vi "Destroy IntelliSenseString.vi"(0 "IntelliSense String":refnum<class "IntelliSenseStringControl.lvclass">, 11 "error in (no error)":errorcluster) -> (15 "error out":errorcluster)   [LabVIEW 2016, in "StringIntelliSense.lvlib"]
uses:
  StringIntelliSense.lvlib
  IntelliSenseStringControl.lvclass
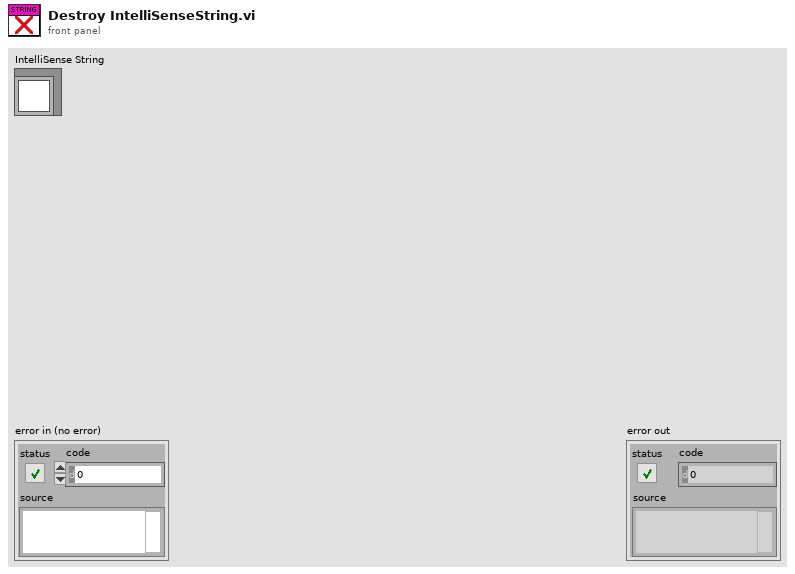
[diagram p1: front panel]
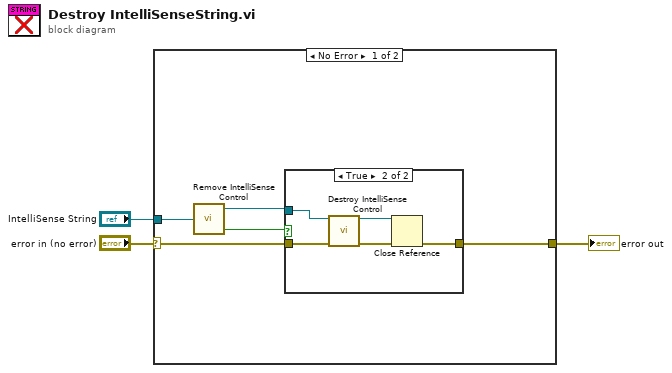
[diagram p0: block diagram]
diagram:
  n1 = case shown="No Error" "error in (no error)" {
    selector: "error in (no error)" -> [w7 w15]
    tunnel: [w8 w15] -> w2
    tunnel: "IntelliSense String" -> [w6 _]
    frame No Error {
      n2 = call "Remove IntelliSense Control.vi"("IntelliSenseStringControl"=w6) -> ("IntelliSenseStringControl"=w5:refnum<class "IntelliSenseStringControl.lvclass">, "removed?"=w4:bool)  [unwired: 1 in]
      n3 = case shown="True" w4 {
        tunnel: [w9 w11] -> w8
        tunnel: w7 -> [w9 w13]
        tunnel: w5 -> [_ w12]
        frame False {
        }
        frame True {
          n4 = call "Destroy IntelliSense Control.vi"("IntelliSense Control"=w12, "error in"=w13) -> ("Str Ctl Refnum"=w10:refnum<vi>, "error out"=w14:errorcluster)  [unwired: 12 in]
          n5 = Close Reference(reference=w10, error in (no error)=w14) -> (error out=w11:errorcluster)
        }
      }
    }
    frame Error {
    }
  }
  "error out" <- w2
